vi "ReadScan2_Rf2.vi"(8 "error in (no error)":errorcluster, 11 "Data In":T3) -> (0 "error out":errorcluster, 1 "Next State":T2=enum."State1", 2 "States":T1, 3 "Data Out":T3)   [LabVIEW 2014]
doc: "Use this template to build a standard state machine design pattern. Each state executes code and determines which state to transition to. Contrast this design pattern with the User Interface Event Handler pattern, in which code executes in response to user actions. Contrast this design pattern also with the Queued Message Handler pattern, in which each message handling code can queue zero or more new messages.\nNote: This template does not contain the most recent programming guidelines recommended by National Instruments. For a complete, project-based implementation of the Standard State Machine pattern, use the Create Project dialog box instead of this template."
uses:
  controls/Data.ctl
  controls/Wait Scan States.ctl
  controls/State.ctl
  controls/ReadScan1States.ctl
panel:
  # "日期"
  # "機種名稱"
  # "機種代號"
  # "商品條碼"
  # "台"
  # "OK"
  # "NG"
  # "台"
  # "總計"
  # "台"
  # "日期"
  # "機種名稱"
  # "機種代號"
  # "商品條碼"
  # "台"
  # "OK"
  # "NG"
  # "台"
  # "總計"
  # "台"
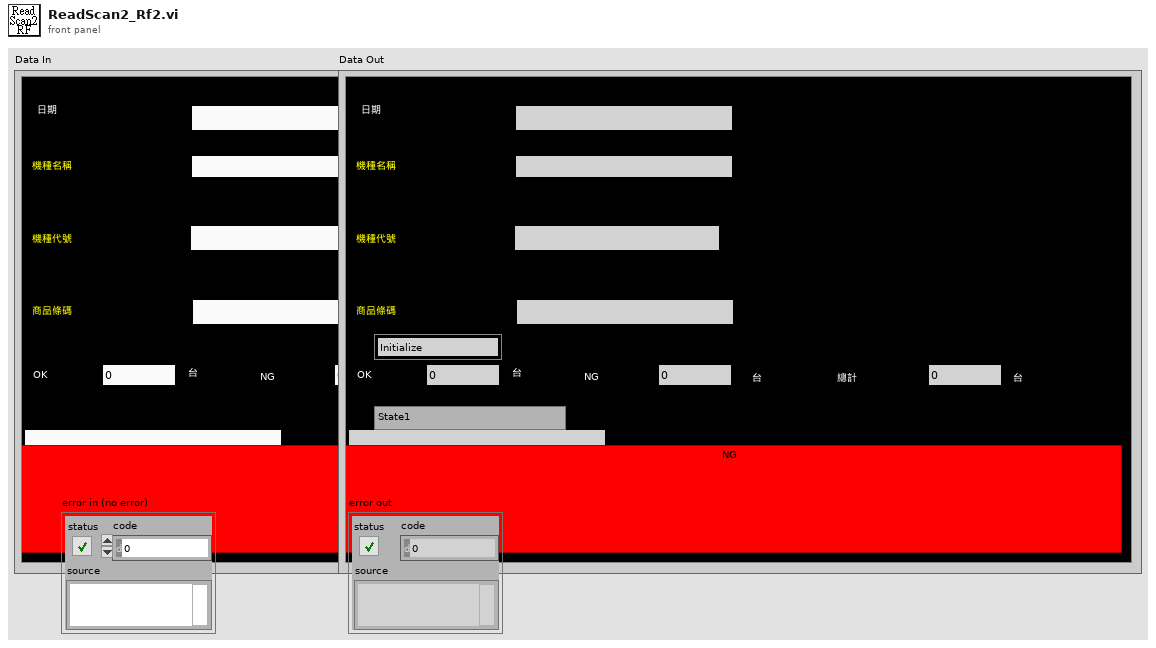
[diagram p1: front panel]
types:
  T1 = typedef "State.ctl" = enum16{"Initialize", "Wait for Scan", "State 1", "State 2", "NG", "NG1", "OK", "OKNG", "Exit"}
  T2 = typedef "Wait Scan States.ctl" = enum16{"Initialize", "State1", "Stop"}
  T3 = typedef "Data.ctl" = cluster{"Date":string, "BarCode1":string, "BarCode2":string, "BarCode3":string, "Message":string, "OK Count":u16, "NG Count":u16, "Total Count":u16, "ModelData":string[][], "OK&NG":bool, "COM1":refnum<visa-resource-name>, "COM2":refnum<visa-resource-name>, "IO":i32, "Time":u32, "TCP":refnum<k5>, "TCP 2":refnum<k5>}
  T4 = typedef "ReadScan1States.ctl" = enum16{"Initialize", "Init2", "Step1", "Step2", "Step3", "Step4", "One", "Two", "Three", "Four", "Five", "End", "Stop"}
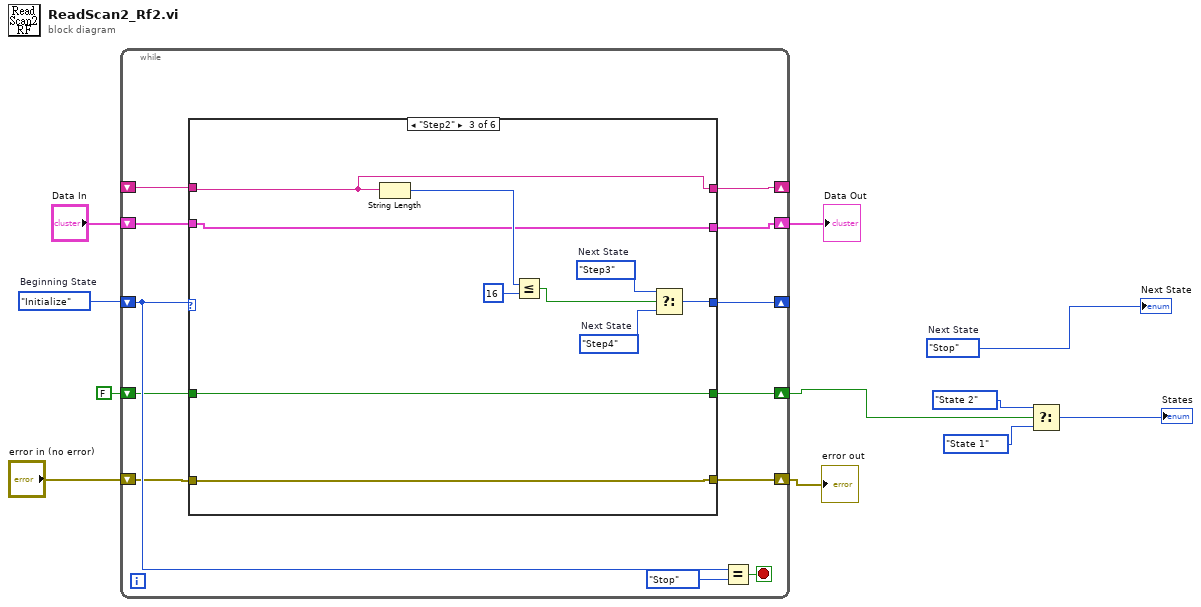
[diagram p0: block diagram]
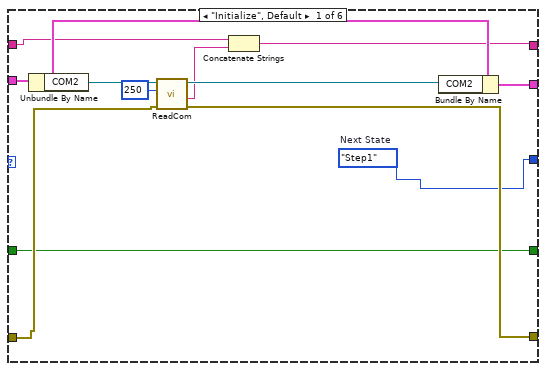
[diagram p2: hidden frame]
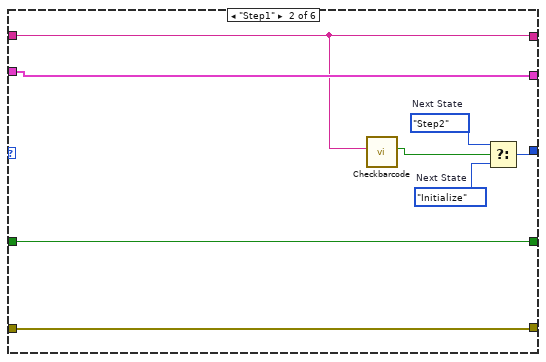
[diagram p3: hidden frame]
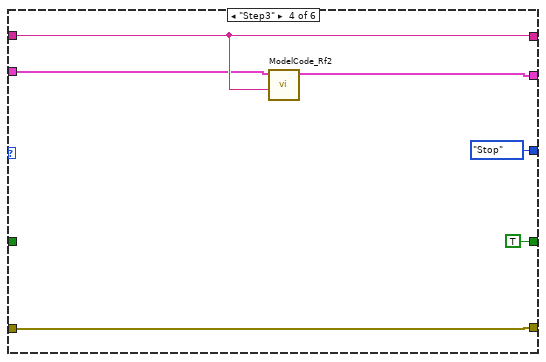
[diagram p4: hidden frame]
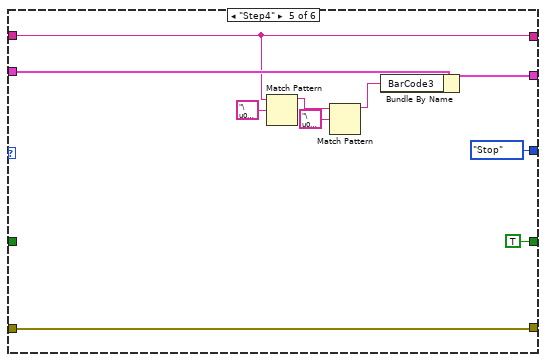
[diagram p5: hidden frame]
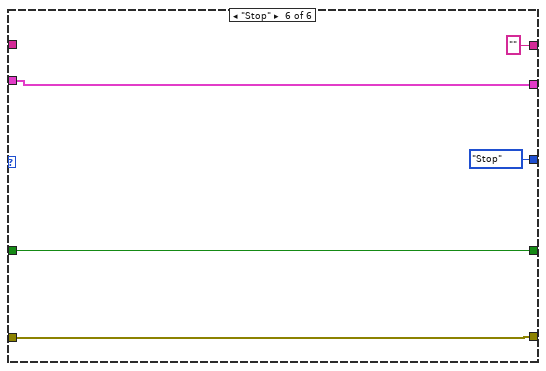
[diagram p6: hidden frame]
diagram:
  w1 = Wait_Scan_States."Stop"  # Next State
  w11 = ReadScan1States."Initialize"  # Beginning State
  n1 = while {
    shift-right: [w20] -> _
    shift-left: w11 -> [w21]
    shift-right: [w15] -> w9
    shift-left: "Data In" -> [w18]
    shift-right: [w14] -> w7
    shift-left: "error in (no error)" -> [w19]
    shift-right: [w16] -> _
    shift-left: _ -> [w17]
    shift-right: [w13] -> w2
    shift-left: FALSE -> [w12]
    stop <- w23 stop-if-true
    n2 = case shown="\"Step2\"" w21 {
      tunnel: [w24 w38 w47 ReadScan1States."Stop" ("Next State") ReadScan1States."Stop" ("Next State") ReadScan1States."Stop" ("Next State")] -> w20
      tunnel: w19 -> [w30 w36 w45 w59 w68 w71]
      tunnel: w18 -> [w33 w43 w51 w56 w67 w72]
      tunnel: w17 -> [w26 w39 w46 w57 w65 _]
      tunnel: [w25 w39 w46 w57 w65 ""] -> w16
      tunnel: [w32 w43 w51 w55 w66 w72] -> w15
      tunnel: [w29 w36 w45 w59 w68 w71] -> w14
      tunnel: [w28 w37 w44 TRUE TRUE w70] -> w13
      tunnel: w12 -> [w28 w37 w44 _ _ w70]
      frame "Initialize", Default {
        w24 = ReadScan1States."Step1"  # Next State
        n3 = Unbundle By Name(w33) -> ("COM2"=w35:refnum<visa-resource-name>)
        n4 = call "ReadCom.vi"("error in (no error)"=w30, "delay before read (ms)"=u32 250, "Com In"=w35) -> ("error out"=w29:errorcluster, "Response"=w27:string, "Com Out"=w31:refnum<visa-resource-name>)  [unwired: 5 in, 1 out]
        n5 = Concatenate Strings(w26, w27) -> (w25:string)
        n6 = Bundle By Name(cluster=w33, "COM2"=w31) -> (w32:T3)
      }
      frame "Step1" {
        w42 = ReadScan1States."Step2"  # Next State
        w41 = ReadScan1States."Initialize"  # Next State
        n7 = call "Checkbarcode.vi"("String In"=w39) -> ("Complete"=w40:bool)  [unwired: 10 in]
        n8 = Select(t=w42, s=w40, f=w41) -> (s? t:f=w38:T4)
      }
      frame "Step2" {
        w50 = ReadScan1States."Step3"  # Next State
        w49 = ReadScan1States."Step4"  # Next State
        n9 = String Length(string=w46) -> (length=w53:i32)
        n10 = Less Or Equal?(x=w53, y=16) -> (x <= y?=w48:bool)
        n11 = Select(t=w50, s=w48, f=w49) -> (s? t:f=w47:T4)
      }
      frame "Step3" {
        n12 = call "ModelCode_Rf2.vi"("BarCode"=w57, "Data In"=w56) -> ("Data Out"=w55:T3)  [unwired: 8 in, 1 out]
      }
      frame "Step4" {
        n13 = Match Pattern(string=w65, regular expression="\u0003") -> (before substring=w63:string)  [unwired: 1 in, 3 out]
        n14 = Match Pattern(string=w63, regular expression="\u0002") -> (before substring=w61:string)  [unwired: 1 in, 3 out]
        n15 = Bundle By Name(cluster=w67, "BarCode3"=w61) -> (w66:T3)
      }
      frame "Stop" {
      }
    }
    n16 = Equal?(x=w21, y=ReadScan1States."Stop" ("States")) -> (x = y?=w23:bool)
  }
  "Data Out" <- w9
  "error out" <- w7
  n17 = Select(t=State."State 2" ("States"), s=w2, f=State."State 1" ("States")) -> (s? t:f=→"States":T1)
  "Next State" <- w1
